vi "Read.vi"(5 "LNAX301":refnum<queue>, 7 "Process":refnum<queue>, 8 "error in (no error)":errorcluster, 10 "Switch Mode":bool, 11 "LNAX301 in":refnum<class "LNAX301.lvclass">) -> (0 "error out":errorcluster, 1 "Data  ok":bool, 2 "Temperature":dbl, 3 "LNAX301 out":refnum<class "LNAX301.lvclass">, 4 "data":i16[](array[numeric]), 6 "OA":i16[][](array[numeric]))   [LabVIEW 2017, in "LNAX301.lvclass"]
uses:
  LNAX301.lvclass
  ModbusRTUCmd.ctl
  Process/Process.ctl
  LNAX301.lvclass/LNAX301.ctl
panel:
  out "time":u32
  out "size(s)":i32
  out "catch time":u32
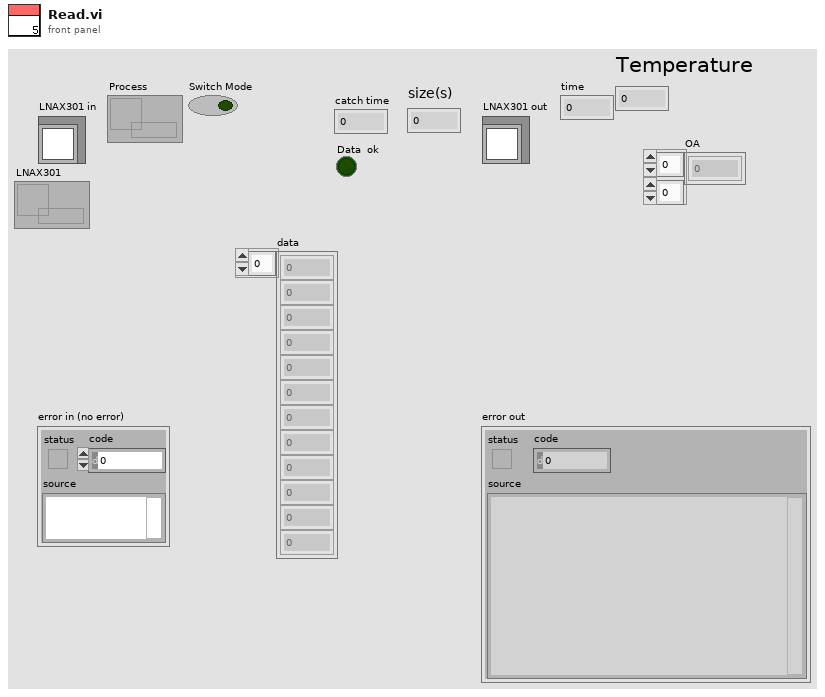
[diagram p1: front panel]
types:
  T1 = typedef "ModbusRTUCmd.ctl" = cluster{"CMD":enum16{"Idle", "ini", "Connect", "Setup", "Read", "Disconnect", "Exit"}, "Var":variant}
  T2 = typedef "Modbus function.ctl" = enum16{"Get Data Length", "Normal Mode", "Bulk Mode"}
  T3 = typedef "ITRI.ctl" = cluster{"amples in buffer":u16, "connect":bool, "CreateRtu":refnum<k24>, "SlaveID":u8, "Com port":string, "data":i16[]}
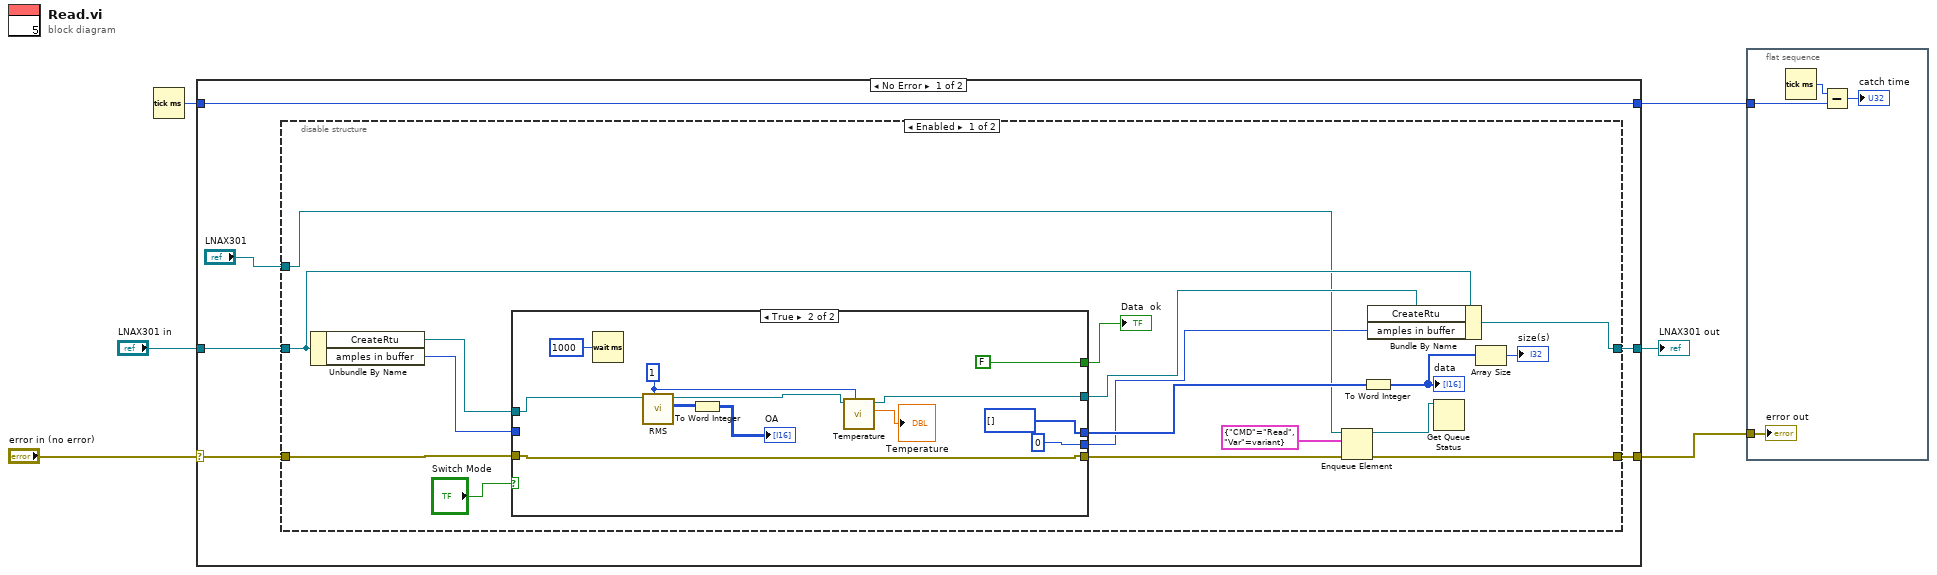
[diagram p0: block diagram]
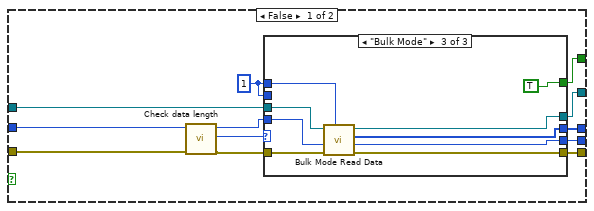
[diagram p2: hidden frame]
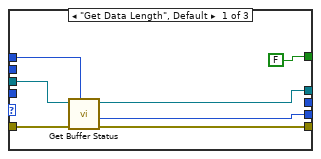
[diagram p3: hidden frame]
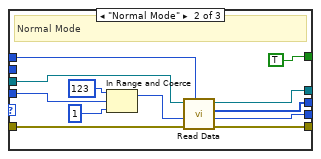
[diagram p4: hidden frame]
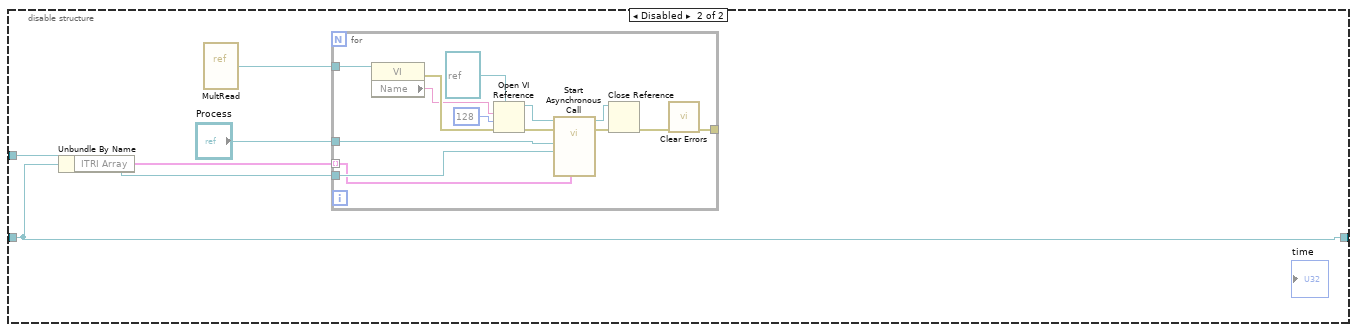
[diagram p5: hidden frame]
diagram:
  n1 = Tick Count (ms)() -> (millisecond timer value=w2:u32)
  n2 = case shown="No Error" "error in (no error)" {
    selector: "error in (no error)" -> [w9 w103]
    tunnel: [w8 w103] -> w5
    tunnel: [w11 w102] -> w3
    tunnel: "LNAX301 in" -> [w12 w102]
    tunnel: w2 -> [w10 w101]
    tunnel: [w10 w101] -> w1
    frame No Error {
      n3 = disable-structure shown="Enabled" {
        disable-tunnel: w12 -> [w29 w86]
        disable-tunnel: [w28 w86] -> w11
        disable-tunnel: w9 -> [w20 _]
        disable-tunnel: [w18 _] -> w8
        disable-tunnel: "LNAX301" -> [w17 w83]
        frame Enabled {
          n4 = Unbundle By Name(w29) -> ("CreateRtu"=w13:refnum<k24>, "amples in buffer"=w16:u16)
          n5 = case shown="True" "Switch Mode" {
            tunnel: [w41 w71] -> w25
            tunnel: [w40 u16[] [] ("Vib")] -> w24
            tunnel: [w39 FALSE] -> w23
            tunnel: w20 -> [w30 w80]
            tunnel: [w38 w80] -> w19
            tunnel: w13 -> [w31 w77]
            tunnel: w16 -> [w33 _]
            tunnel: [w32 u16 0 ("# samples in buffer")] -> w15
            frame False {
              w34 = u8 1 ("SlaveID")
              n6 = call "Check data length.vi"("error in"=w30, "# samples in buffer"=w33) -> ("error out"=w35:errorcluster, "Modbus Function"=w36:T2, "# samples in buffer out"=w37:u16)  [unwired: 7 in]
              n7 = case shown="\"Bulk Mode\"" w36 {
                tunnel: w31 -> [w47 w60 w69]
                tunnel: [w45 w59 w67] -> w38
                tunnel: w37 -> [_ w50 w64]
                tunnel: w34 -> [w42 w58 w65]
                tunnel: [w46 w57 w66] -> w41
                tunnel: w35 -> [w44 w56 w68]
                tunnel: [_ w55 w63] -> w40
                tunnel: [FALSE TRUE TRUE] -> w39
                tunnel: [w43 w49 w61] -> w32
                tunnel: w34 -> [_ _ _]
                frame "Get Data Length", Default {
                  n8 = call "Get Buffer Status.vi"("SlaveID"=w42, "error in (no error)"=w44, ".NET Refnum in"=w47) -> ("error out"=w45:errorcluster, "# samples in buffer"=w43:u16, ".NET Refnum out"=w46:refnum<k24>)  [unwired: 5 in, 1 out]
                }
                frame "Normal Mode" {
                  # "Normal Mode"
                  n9 = In Range and Coerce(upper limit=u16 123, x=w50, lower limit=u16 1) -> (coerced(x)=w51:u16)  [unwired: 1 out]
                  n10 = call "Read Data.vi"("SlaveID"=w58, "error in (no error)"=w56, "# samples to read"=w51, ".NET Refnum in"=w60) -> ("error out"=w59:errorcluster, "# samples in buffer"=w49:u16, "Vib"=w55:u16[], "reference out"=w57:refnum<k24>)  [unwired: 4 in]
                }
                frame "Bulk Mode" {
                  n11 = call "Bulk Mode Read Data.vi"("SlaveID"=w65, "error in (no error)"=w68, "# samples to read"=w64, ".NET Refnum in"=w69) -> ("error out"=w67:errorcluster, "# samples in buffer"=w61:u16, "Vib"=w63:u16[], "reference out"=w66:refnum<k24>)  [unwired: 4 in]
                }
              }
            }
            frame True {
              w72 = u8 1 ("SlaveID")
              n12 = Wait (ms)(milliseconds to wait=u32 1000) -> ()  [unwired: 1 out]
              n13 = call "RMS.vi"("SlaveID"=w72, ".NET Refnum in"=w77) -> ("OA"=w78:u16[][], "reference out"=w73:refnum<k24>)  [unwired: 7 in, 1 out]
              n14 = To Word Integer(number=w78) -> (16bit integer=→"OA":i16[][])
              n15 = call "Temperature.vi"("SlaveID"=w72, ".NET Refnum in"=w73) -> ("Temperature"=→"Temperature":dbl, "reference out"=w71:refnum<k24>)  [unwired: 7 in, 1 out]
            }
          }
          "Data  ok" <- w23
          n16 = Enqueue Element(queue=w17, element=T1 {"CMD"=enum."Read", "Var"=variant}, error in (no error)=w19) -> (queue out=w26:refnum<queue>, error out=w18:errorcluster)  [unwired: 1 in, 1 out]
          n17 = To Word Integer(number=w24) -> (16bit integer=w22:i16[])
          "data" <- w22
          n18 = Bundle By Name(cluster=w29, "CreateRtu"=w25, "amples in buffer"=w15) -> (w28:refnum<class "LNAX301.lvclass">)
          n19 = Get Queue Status(queue=w26) -> ()  [unwired: 2 in, 8 out]
          n20 = Array Size(array=w22) -> (size(s)=→"size(s)":i32)
        }
        frame Disabled {
          n21 = Unbundle By Name(w86) -> ("ITRI Array"=w82:T3[])
          n22 = vi-ref "MultRead.vi"() -> (w85:refnum<vi>)
          n23 = for {
            tunnel: w82 -> [w87] mode=indexing
            tunnel: w85 -> [w95]
            tunnel: [w90] -> _
            tunnel: "Process" -> [w89]
            tunnel: w83 -> [w88]
            n24 = property class="VI"(reference=w95) -> (error out=w99:errorcluster, "Name"=w98:string)  [unwired: 1 in, 1 out]
            n25 = Open VI Reference(type specifier VI Refnum (for type only)=refnum<vi> refnum, vi path=w98, options=128, error in (no error)=w99) -> (vi reference=w97:refnum<vi>, error out=w96:errorcluster)  [unwired: 2 in]
            n26 = call-by-ref "Start Asynchronous Call"(reference=w97, error in=w96, "ITRI"=w87, "LNAX301"=w88, "Process"=w89) -> (reference out=w93:refnum<vi>, error out=w92:errorcluster)  [unwired: 8 in, 1 out]
            n27 = Close Reference(reference=w93, error in (no error)=w92) -> (error out=w91:errorcluster)
            n28 = call <vilib>:"Clear Errors.vi"("error in (no error)"=w91) -> ("error out"=w90:errorcluster)  [unwired: 5 in, 1 out]
          }
        }
      }
    }
    frame Error {
    }
  }
  "LNAX301 out" <- w3
  n29 = flat-sequence {
    tunnel: w5 -> [w107]
    tunnel: w1 -> [w104]
    frame #0 {
      n30 = Tick Count (ms)() -> (millisecond timer value=w105:u32)
      n31 = Subtract(x=w105, y=w104) -> (x-y=→"catch time":u32)
      "error out" <- w107
    }
  }
